vi "Main-Calculate PSD by ACF or direct FFT-v2.vi"() -> ()   [LabVIEW 2014]
uses:
  <vilib>/Analysis/2dsp.llb/Real FFT.vi
  <vilib>/Utility/file.llb/Read From Spreadsheet File (DBL).vi
  <vilib>/Analysis/NI_AALBase.lvlib
  <vilib>/Analysis/NI_AALPro.lvlib
panel:
  out "Fs":dbl
  out "Avg. Array":dbl[](array[numeric])
  out "X":dbl[][](array[numeric])
  out "ACF":dbl[][](array[numeric])
  in  "# of avg":i32
  out "df":dbl
  in  "ACF length":i32=2130
  in  "Filter?":bool
  in  "left rank":i32=2
  in  "Tab Control":enum32{"Page 1", "Page 2", "Acg. ACF", "Page 4"}(tab)
  out "Waveform Graph":dbl[](graph)
  out "XY Graph":T1(graph)
  out "XY Graph 2":cluster{"Avg. Array":dbl[], "Avg. Array":dbl[]}(graph)
  out "XY Graph 3":cluster{"Avg. Array":dbl[], "Avg. Array":dbl[]}(graph)
  out "Fs":dbl
  in  "intervals":i32=5000
  in  "T=ACF method\nF=direct FT method":bool
  in  "file path (dialog if empty)":path=path "D:/OneDrive - g.ntu.edu.tw/OT/OT data/可用data---/pFC-mRad51 assembly/twoday.txt"
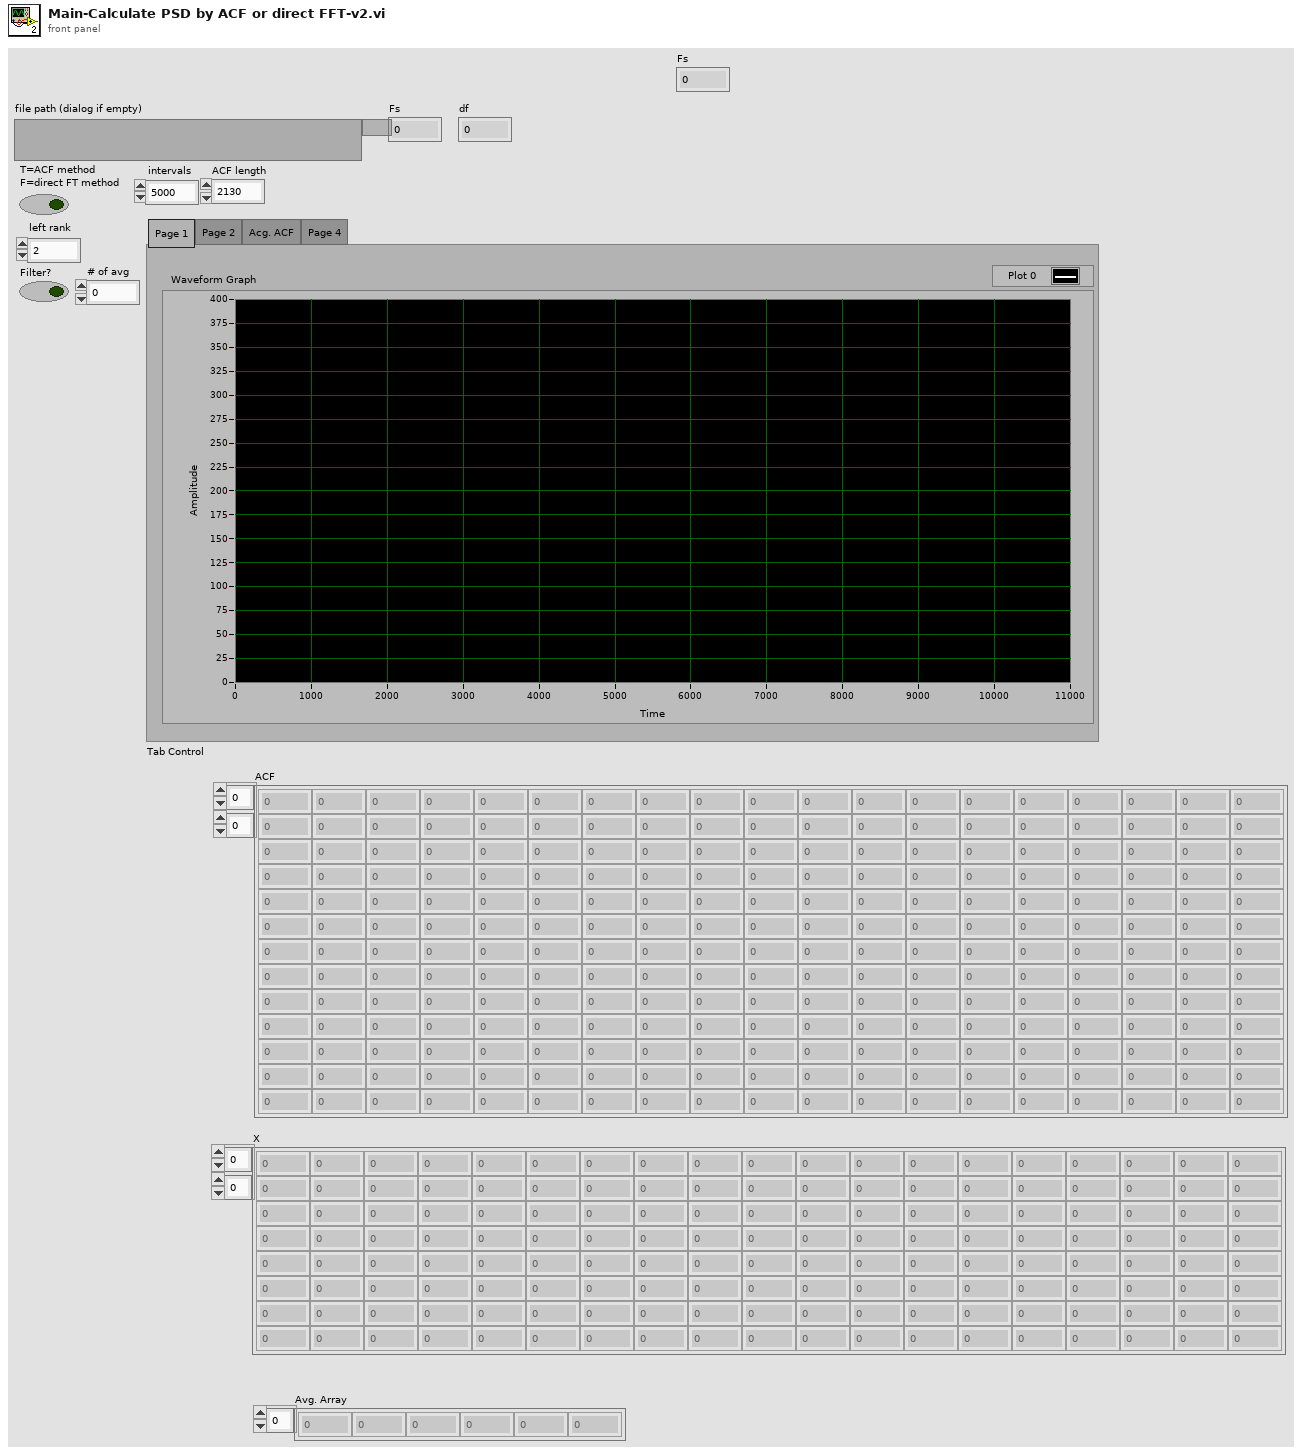
[diagram p1: front panel]
types:
  T1 = cluster{"Frequency,0 df,2df,...,(Hz)":dbl[], "PSD":dbl[]}
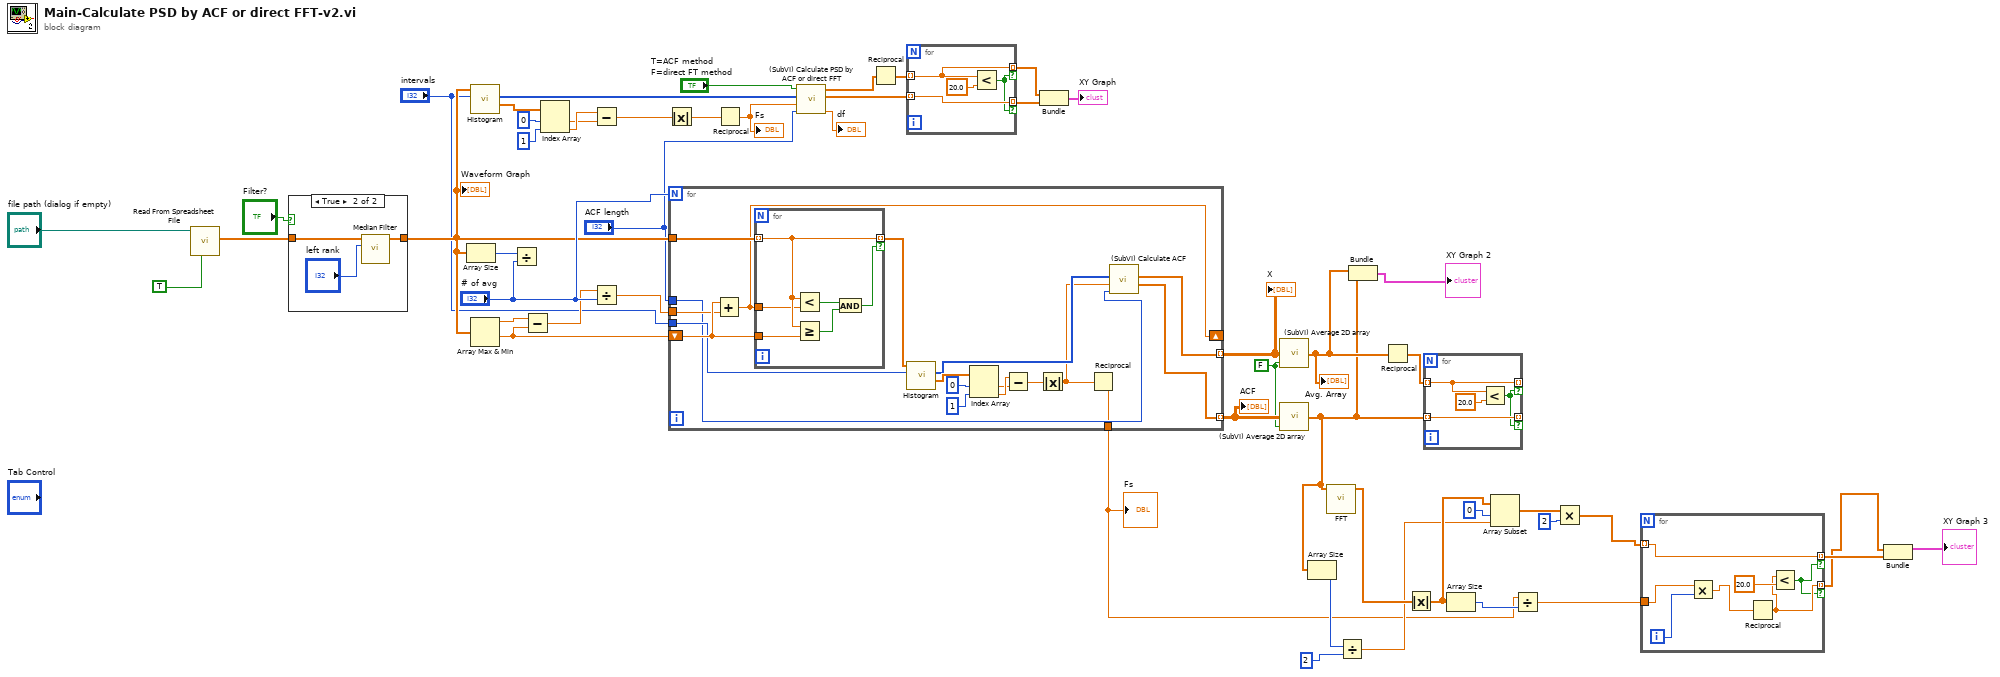
[diagram p0: block diagram]
diagram:
  w22 = FALSE ("Transpose?")
  n1 = call-poly <vilib>:"Read From Spreadsheet File.vi"("transpose (no:F)"=TRUE, "file path (dialog if empty)"="file path (dialog if empty)") -> ("first row"=w38:dbl[])  [unwired: 5 in, 4 out]
  n2 = case shown="True" "Filter?" {
    tunnel: w38 -> [w53 w56]
    tunnel: [w53 w55] -> w27
    frame False {
    }
    frame True {
      n3 = call <vilib>:"Median Filter.vi"("left rank"="left rank", "X"=w56) -> ("Filtered X"=w55:dbl[])  [unwired: 8 in, 1 out]
    }
  }
  "Waveform Graph" <- w27
  n4 = Array Size(array=w27) -> (size(s)=w31:i32)
  n5 = call <vilib>:"Histogram.vi"("intervals"="intervals", "X"=w27) -> ("X Values"=w49:dbl[], "Histogram: h(x)"=w41:i32[])  [unwired: 6 in, 2 out]
  n6 = Array Max & Min(array=w27) -> (max value=w30:dbl, min value=w26:dbl)  [unwired: 2 out]
  n7 = Divide(x=w31, y="# of avg") -> ()  [unwired: 1 out]
  n8 = Subtract(x=w30, y=w26) -> (x-y=w28:dbl)
  n9 = Index Array(array=w49, index #1=0 ("index"), index #2=1 ("index")) -> (element #1=w45:dbl, element #2=w46:dbl)
  n10 = Subtract(x=w46, y=w45) -> (x-y=w44:dbl)
  n11 = Divide(x=w28, y="# of avg") -> (x/y=w25:dbl)
  n12 = Absolute Value(x=w44) -> (abs(x)=w43:dbl)
  n13 = for {
    N: "# of avg" -> [_]
    tunnel: w27 -> [w74]
    tunnel: w25 -> [w71]
    shift-right: [w70] -> _
    shift-left: w26 -> [w73]
    tunnel: "ACF length" -> [w60]
    tunnel: [w58] -> w24 mode=indexing
    tunnel: [w59] -> w23 mode=indexing
    tunnel: "intervals" -> [w69]
    tunnel: [w57] -> w5
    n14 = Add(x=w73, y=w71) -> (x+y=w70:dbl)
    n15 = for {
      tunnel: w74 -> [w80] mode=indexing
      tunnel: [w80] -> w72 mode=indexing if=w77
      tunnel: w73 -> [w76]
      tunnel: w70 -> [w75]
      n16 = Less?(x=w80, y=w75) -> (x < y?=w79:bool)
      n17 = Greater Or Equal?(x=w80, y=w76) -> (x >= y?=w78:bool)
      n18 = And(x=w79, y=w78) -> (x .and. y?=w77:bool)
    }
    n19 = call <vilib>:"Histogram.vi"("intervals"=w69, "X"=w72) -> ("X Values"=w63:dbl[], "Histogram: h(x)"=w62:i32[])  [unwired: 6 in, 2 out]
    n20 = Index Array(array=w63, index #1=0 ("index"), index #2=1 ("index")) -> (element #1=w65:dbl, element #2=w66:dbl)
    n21 = Subtract(x=w66, y=w65) -> (x-y=w64:dbl)
    n22 = Absolute Value(x=w64) -> (abs(x)=w61:dbl)
    n23 = Reciprocal(x=w61) -> (1/x=w57:dbl)
    n24 = call "(SubVI) Calculate ACF .vi"("ACF length"=w60, "dt"=w61, "Data"=w62) -> ("ACF"=w58:dbl[], "x or t"=w59:dbl[])  [unwired: 3 in]
  }
  "ACF" <- w24
  "X" <- w23
  "Fs" <- w5
  n25 = Reciprocal(x=w43) -> (1/x=w42:dbl)
  "Fs" <- w42
  n26 = call "(SubVI) Calculate PSD by ACF or direct FFT.vi"("ACF length"="ACF length", "Fs"=w42, "Data"=w41, "T=ACF method\nF=direct FT method"="T=ACF method\nF=direct FT method") -> ("df"=→"df":dbl, "PSD"=w35:dbl[], "Frequency,0 df,2df,...,(Hz)"=w39:dbl[])  [unwired: 2 in, 1 out]
  n27 = Reciprocal(x=w39) -> (1/x=w36:dbl[])
  n28 = for {
    tunnel: w36 -> [w83] mode=indexing
    tunnel: w35 -> [w82] mode=indexing
    tunnel: [w83] -> w33 mode=indexing if=w81
    tunnel: [w82] -> w34 mode=indexing if=w81
    n29 = Less?(x=w83, y=20.0) -> (x < y?=w81:bool)
  }
  n30 = Bundle(w33, w34) -> (→"XY Graph":cluster{dbl[], dbl[]})  [unwired: 1 in]
  n31 = call "(SubVI) Average 2D array.vi"("Transpose?"=w22, "Array"=w23) -> ("Avg. Array"=w18:dbl[])  [unwired: 3 in]
  "Avg. Array" <- w18
  n32 = call "(SubVI) Average 2D array.vi"("Transpose?"=w22, "Array"=w24) -> ("Avg. Array"=w10:dbl[])  [unwired: 3 in]
  n33 = Array Size(array=w10) -> (size(s)=w9:i32)
  n34 = call-poly <vilib>:"FFT.vi"("X"=w10) -> ("FFT {X}"=w11:cdb[])  [unwired: 9 in, 1 out]
  n35 = Divide(x=w9, y=2 ("index")) -> (x/y=w7:dbl)
  n36 = Bundle("Avg. Array"=w18, "Avg. Array"=w10) -> (→"XY Graph 2":cluster{"Avg. Array":dbl[], "Avg. Array":dbl[]})  [unwired: 1 in]
  n37 = Reciprocal(x=w18) -> (1/x=w21:dbl[])
  n38 = Absolute Value(x=w11) -> (abs(x)=w12:dbl[])
  n39 = for {
    tunnel: w21 -> [w87] mode=indexing
    tunnel: w10 -> [w86] mode=indexing
    tunnel: [w87] -> _ mode=indexing if=w85
    tunnel: [w86] -> _ mode=indexing if=w85
    n40 = Less?(x=w87, y=20.0) -> (x < y?=w85:bool)
  }
  n41 = Array Size(array=w12) -> (size(s)=w6:i32)
  n42 = Array Subset(array=w12, index=0, length=w7) -> (w14:dbl[])
  n43 = Divide(x=w5, y=w6) -> (x/y=w3:dbl)
  n44 = Multiply(x=w14, y=2) -> (x*y=w4:dbl[])
  n45 = for {
    tunnel: w4 -> [w93] mode=indexing
    tunnel: w3 -> [w94]
    tunnel: [w90] -> w1 mode=indexing if=w89
    tunnel: [w93] -> w2 mode=indexing if=w89
    i -> [w95]
    n46 = Multiply(x=w94, y=w95) -> (x*y=w92:dbl)
    n47 = Reciprocal(x=w92) -> (1/x=w90:dbl)
    n48 = Less?(x=w90, y=20.0) -> (x < y?=w89:bool)
  }
  n49 = Bundle(w1, w2) -> (→"XY Graph 3":cluster{dbl[], dbl[]})  [unwired: 1 in]
